vi "Read Variable.vi"(8 "error in (no error)":errorcluster, 10 "PG path":string, 11 "Data.PGQL in":refnum<class "Data.PGSQL.lvclass">) -> (0 "error out":errorcluster, 1 "Time Stamp":timestamp, 2 "Value":dbl, 3 "Data.PGSQL out":refnum<class "Data.PGSQL.lvclass">, 4 "Column (units)":string)   [LabVIEW 2013, in "Data.PGSQL.lvclass"]
uses:
  Data.PGSQL.lvclass
panel:
  out "resulting string":string
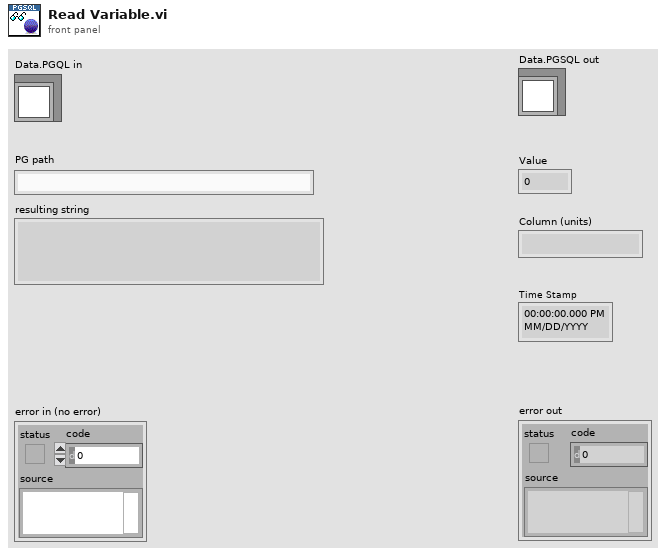
[diagram p1: front panel]
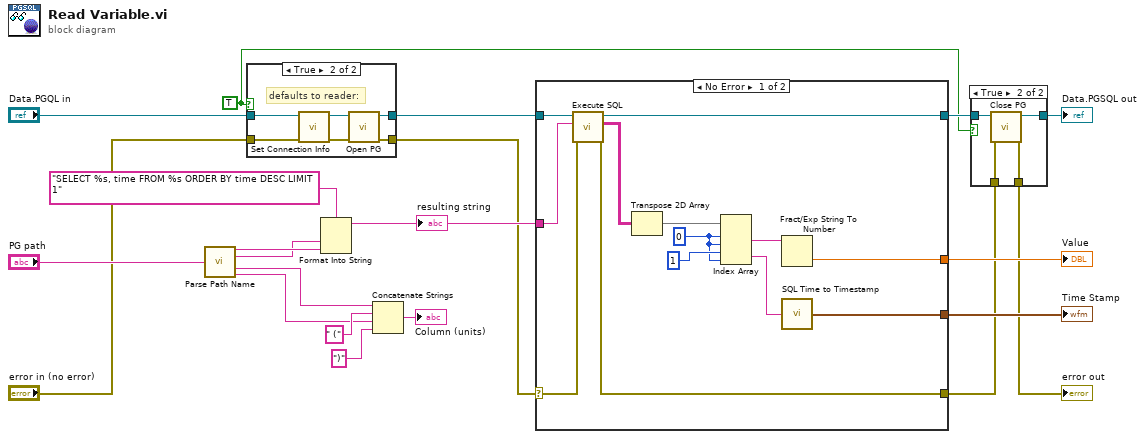
[diagram p0: block diagram]
diagram:
  w1 = TRUE
  n1 = call "Parse Path Name.vi"("PG Path"="PG path") -> ("Table path"=w18:string, "Column path"=w17:string, "Column name"=w12:string, "Column units"=w13:string)  [unwired: 10 in, 1 out]
  n2 = case shown="True" w1 {
    tunnel: "Data.PGQL in" -> [w23 w29]
    tunnel: "error in (no error)" -> [w22 w28]
    tunnel: [w23 w25] -> w7
    tunnel: [w22 w24] -> w6
    frame False {
    }
    frame True {
      # "defaults to reader:"
      n3 = call "Set Connection Info.vi"("Data.PG in"=w29, "error in (no error)"=w28) -> ("Data.PG out"=w27:refnum<class "Data.PGSQL.lvclass">, "error out"=w26:errorcluster)  [unwired: 7 in]
      n4 = call-dynamic "Open PG.vi"("error in (no error)"=w26, "Data.PG in"=w27) -> ("error out"=w24:errorcluster, "Data.PG out"=w25:refnum<class "Data.PGSQL.lvclass">)  [unwired: 8 in]
    }
  }
  n5 = Format Into String(format string="SELECT %s, time FROM %s ORDER BY time DESC LIMIT 1", w17, w18) -> (resulting string=w15:string)  [unwired: 2 in, 1 out]
  "resulting string" <- w15
  n6 = Concatenate Strings(w12, " (" ("string"), w13, ")" ("string")) -> (→"Column (units)":string)
  n7 = case shown="No Error" w6 {
    selector: w6 -> [w36 w43]
    tunnel: w7 -> [w41 w44]
    tunnel: w15 -> [w38 _]
    tunnel: [w40 w43] -> w3
    tunnel: [w39 w44] -> w5
    tunnel: [w33 _] -> w11
    tunnel: [w32 _] -> w10
    frame No Error {
      w30 = 0 ("index (row)")
      n8 = call "Execute SQL.vi"("error in"=w36, "SQL"=w38, "Data.PG"=w41) -> ("error out"=w40:errorcluster, "Result"=w37:string[][], "Data.PG out"=w39:refnum<class "Data.PGSQL.lvclass">)  [unwired: 6 in]
      n9 = Transpose 2D Array(2D array=w37) -> (transposed array=w42:string[][])
      n10 = Index Array(array=w42, index (row) #1=w30, index (col) #1=w30, index (row) #2=1 ("index (row)"), index (col) #2=w30) -> (element #1=w35:string, element #2=w34:string)
      n11 = Fract/Exp String To Number(string=w35) -> (number=w33:dbl)  [unwired: 3 in, 1 out]
      n12 = call "SQL Time to Timestamp.vi"("Get:Get String"=w34) -> ("Time Stamp"=w32:timestamp)
    }
    frame Error {
    }
  }
  "Time Stamp" <- w10
  "Value" <- w11
  n13 = case shown="True" w1 {
    tunnel: w5 -> [w46 w50]
    tunnel: [w46 w49] -> w4
    tunnel: w3 -> [w45 w48]
    tunnel: [w45 w47] -> w2
    frame False {
    }
    frame True {
      n14 = call-dynamic "Close PG.vi"("error in (no error)"=w48, "Data.PG in"=w50) -> ("error out"=w47:errorcluster, "Data.PG out"=w49:refnum<class "Data.PGSQL.lvclass">)  [unwired: 8 in]
    }
  }
  "error out" <- w2
  "Data.PGSQL out" <- w4
